vi "JSON Array to Array of JSON Strings.vi"(11 "JSON Array Value":string="[{\"Numeric\":121,\"Boolean\":false,\"Enum\":\"first\",\"Path\":\"C:\\test\",\"String\":\"examplestring\"},{\"Numeric\":121,\"Boolean\":true,\"Enum\":\"second\",\"Path\":\"D:\\stest\",\"String\":\"asdfasd\"}]") -> (3 "Array of JSON Values":string[](array[string]), 5 "JSON Value Type":T1)   [LabVIEW 2011, in "LV JSON.lvlib"]
uses:
  LV JSON.lvlib
  controls/JSON type.ctl
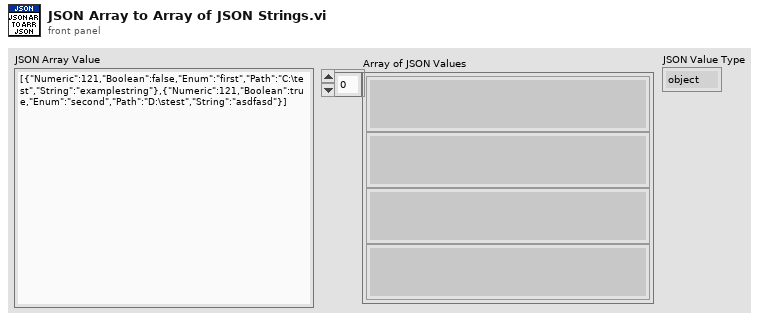
[diagram p1: front panel]
types:
  T1 = typedef "LV JSON.lvlib/JSON type.ctl" = enum16{"object", "array", "number", "string", "boolean", "null"}
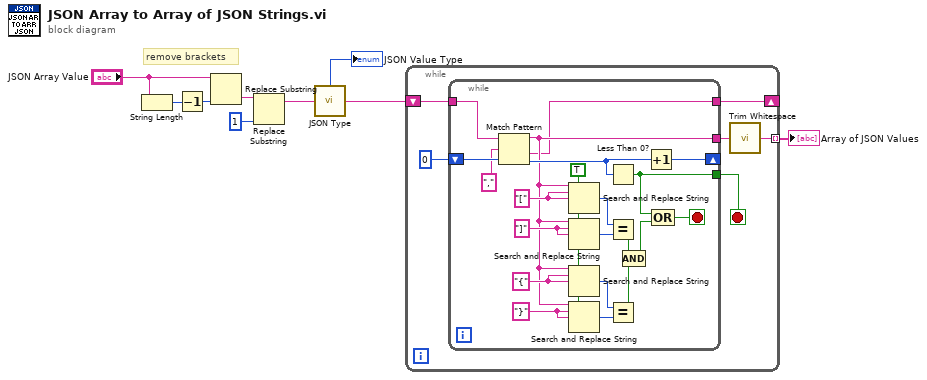
[diagram p0: block diagram]
diagram:
  # "remove brackets"
  n1 = String Length(string="JSON Array Value") -> (length=w7:i32)
  n2 = Decrement(x=w7) -> (x-1=w8:i32)
  n3 = Replace Substring(2:w8, 5:"JSON Array Value") -> (0:w9:string)  [unwired: 2 in, 1 out]
  n4 = Replace Substring(2:1 ("length (len. of substring)"), 5:w9) -> (1:w3:string)  [unwired: 2 in, 1 out]
  n5 = call "JSON Type.vi"("JSON Value"=w3) -> ("JSON Value Type"=→"JSON Value Type":T1, "JSON Value Out (dup)"=w2:string)
  n6 = while {
    tunnel: [w10] -> w4 mode=indexing
    shift-right: [w13] -> _
    shift-left: w2 -> [w12]
    stop <- w14 stop-if-true
    n7 = while {
      tunnel: w12 -> [w33]
      shift-right: [w30] -> _
      shift-left: 0 -> [w32]
      tunnel: [w23] -> w15
      tunnel: [w18] -> w14
      tunnel: [w16] -> w13
      stop <- w34 stop-if-true
      w27 = "}" ("search string")
      w26 = "{" ("replace string (\"\")")
      w28 = "]" ("search string")
      w29 = "[" ("replace string (\"\")")
      w22 = TRUE ("replace all? (F)")
      n8 = Match Pattern(string=w33, regular expression="," ("search string/char (-)"), offset (0)=w32) -> (before substring=w23:string, after substring=w16:string, offset past match=w31:i32)  [unwired: 1 out]
      n9 = Search and Replace String(replace all?=w22, input string=w23, search string=w29, replace string=w29) -> (number of replacements=w35:i32)  [unwired: 4 in, 3 out]
      n10 = Search and Replace String(replace all?=w22, input string=w23, search string=w28, replace string=w28) -> (number of replacements=w36:i32)  [unwired: 4 in, 3 out]
      n11 = Search and Replace String(replace all?=w22, input string=w23, search string=w26, replace string=w26) -> (number of replacements=w25:i32)  [unwired: 4 in, 3 out]
      n12 = Search and Replace String(replace all?=w22, input string=w23, search string=w27, replace string=w27) -> (number of replacements=w24:i32)  [unwired: 4 in, 3 out]
      n13 = Less Than 0?(x=w31) -> (x < 0?=w18:bool)
      n14 = Equal?(x=w35, y=w36) -> (x = y?=w20:bool)
      n15 = Equal?(x=w25, y=w24) -> (x = y?=w19:bool)
      n16 = Compound Arithmetic op=AND(w20, w19) -> (w21:bool)
      n17 = Increment(x=w31) -> (x+1=w30:i32)
      n18 = Compound Arithmetic op=OR(w18, w21) -> (w34:bool)
    }
    n19 = call <vilib>:"Trim Whitespace.vi"("string"=w15) -> ("trimmed string"=w10:string)  [unwired: 1 in]
  }
  "Array of JSON Values" <- w4
